vi "User prompt start IviumSoft.vi"(0 "Enable":bool=TRUE, 5 "error in (no error)":errorcluster) -> (18 "OK":bool, 19 "error out":errorcluster)   [LabVIEW 2020]
doc: "Displays a standard dialog box that prompts users to enter information, such as a user name and password.\n--------------------\n\nThis Express VI is configured as follows:\n\nMessage to Display to the User:Please, start IviumSoft before running this VI\nThe inputs are:"
panel:
  out "String":string="Please, start IviumSoft before running this VI"
  in  "Cancel":bool
  in  "OK2":bool
  in  "OK1":bool
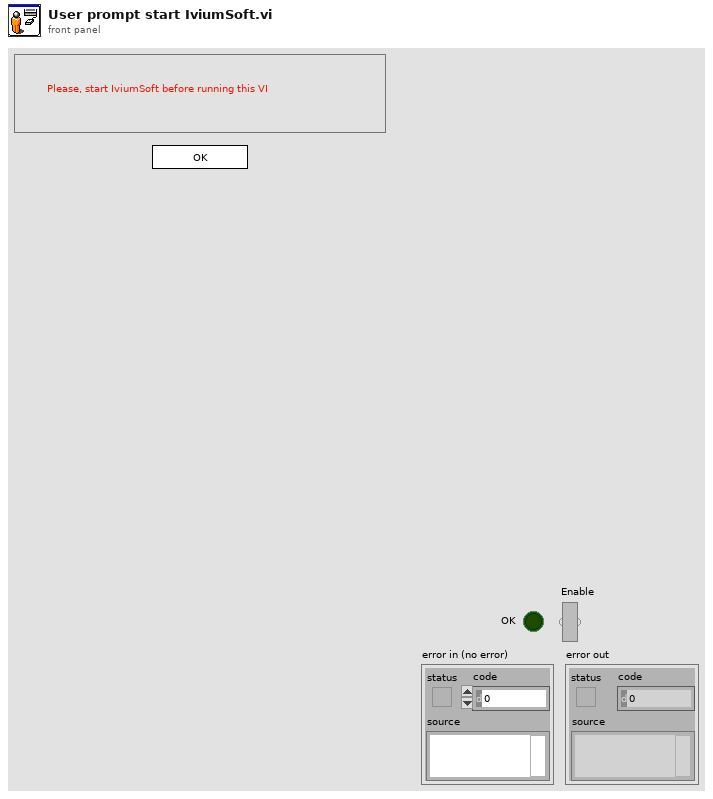
[diagram p1: front panel]
types:
  T1 = cluster{"Input Name":string, "Input Data Type":i32}[]
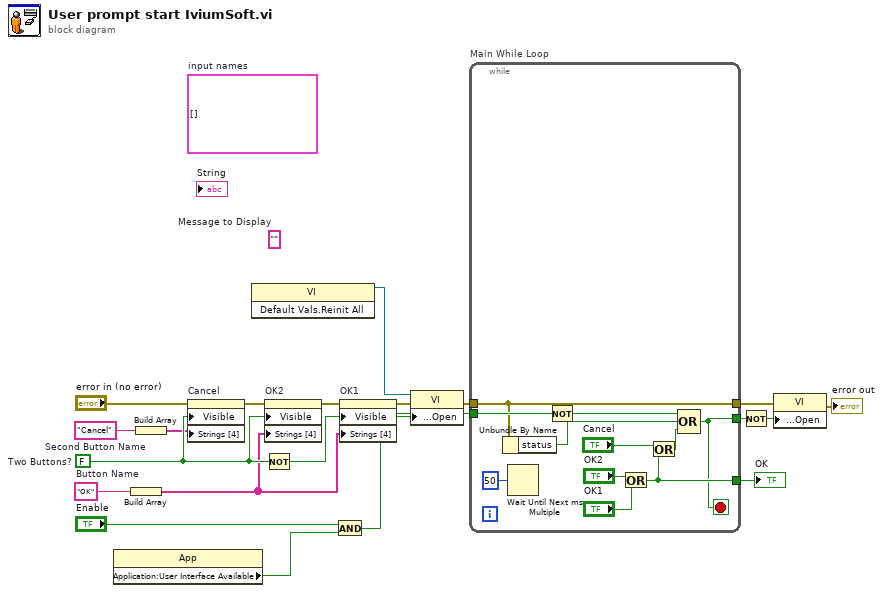
[diagram p0: block diagram]
diagram:
  (unwired) T1 []  # input names
  w12 = "Cancel"  # Second Button Name
  w10 = "OK"  # Button Name
  (unwired) ""  # Message to Display
  w20 = FALSE  # Two Buttons?
  n1 = property class="App"() -> ("Application:User Interface Available"=w2:bool)  [unwired: 2 in, 2 out]
  n2 = Build Array(w10) -> (w11:string[])
  n3 = Build Array(w12) -> (w13:string[])
  n4 = property on="Cancel" class="Bool"(error in="error in (no error)", "Visible"=w20, "Strings [4]"=w13) -> (error out=w17:errorcluster)  [unwired: 1 in, 1 out]
  n5 = invoke class="VI" method="Default Vals.Reinit All"() -> (reference out=w1:refnum<vi>)  [unwired: 3 in, 2 out]
  n6 = Not(x=w20) -> (.not. x?=w18:bool)
  n7 = property on="OK2" class="Bool"(error in=w17, "Visible"=w20, "Strings [4]"=w11) -> (error out=w16:errorcluster)  [unwired: 1 in, 1 out]
  n8 = And(x="Enable", y=w2) -> (x .and. y?=w3:bool)
  n9 = property on="OK1" class="Bool"(error in=w16, "Visible"=w18, "Strings [4]"=w11) -> (error out=w9:errorcluster)  [unwired: 1 in, 1 out]
  n10 = property class="VI"(reference=w1, error in=w9, "Front Panel Window:Open"=w3) -> (error out=w8:errorcluster)  [unwired: 1 out]
  n11 = while "Main While Loop" {
    tunnel: [w28] -> w19
    tunnel: w3 -> [w26]
    tunnel: [w24] -> w14
    tunnel: w8 -> [w23]
    tunnel: [w23] -> w6
    stop <- w24 stop-if-true
    n12 = Unbundle By Name(w23) -> ("status"=w21:bool)
    n13 = Wait Until Next ms Multiple(millisecond multiple=u32 50) -> ()  [unwired: 1 out]
    n14 = Not(x=w26) -> (.not. x?=w25:bool)
    n15 = Or(x="OK2", y="OK1") -> (x .or. y?=w28:bool)
    n16 = Or(x="Cancel", y=w28) -> (x .or. y?=w22:bool)
    n17 = Compound Arithmetic op=OR(w25, w21, w22) -> (w24:bool)
  }
  "OK" <- w19
  n18 = Not(x=w14) -> (.not. x?=w15:bool)
  n19 = property class="VI"(error in=w6, "Front Panel Window:Open"=w15) -> (error out=→"error out":errorcluster)  [unwired: 1 in, 1 out]
